vi "MNIST_Classifier_MLP(Train).vi.vi"() -> ()   [LabVIEW 2024]
doc: "This example demonstrating the usage of Deep Learning Toolkit for solving hand written digit recognition problem with multilayer perceptron (MLP).\nDataset: MNIST http://yann.lecun.com/exdb/mnist/\nRequirements: Deep Learning Toolkit for LabVIEW.s"
uses:
  <vilib>/Ngene/Deep Learning Toolkit/Toolkit/NN_Train/Controls/NN_Train_Params.ctl
  <vilib>/Ngene/Deep Learning Toolkit/Toolkit/NN_Train/Controls/NN_Train_Optimizer.ctl
  <vilib>/Ngene/Deep Learning Toolkit/Toolkit/NN_Train/Controls/NN_Train_Data_Sampling.ctl
  _Controls/Img_GrayScale.ctl
  <vilib>/Ngene/Deep Learning Toolkit/Toolkit/NN_Train/Controls/NN_Train_Session_Data.ctl
  <vilib>/Ngene/Deep Learning Toolkit/Toolkit/NN_Train/Controls/NN_LR_Policy_Cfg.ctl
  <vilib>/Ngene/Deep Learning Toolkit/Toolkit/NN_Train/Controls/NN_LR_Policy_Type.ctl
  <vilib>/Ngene/Deep Learning Toolkit/Toolkit/NN_Network/Controls/NN_Device.ctl
  <vilib>/Ngene/Deep Learning Toolkit/Toolkit/NN_Layers/Layers/FC/Controls/NN_Layer_Config(FC).ctl
  <vilib>/Ngene/Deep Learning Toolkit/Toolkit/NN_Layers/Layers/BatchNorm/Controls/NN_BN_Params.ctl
  <vilib>/Ngene/Deep Learning Toolkit/Toolkit/NN_Activations/Controls/NN_Activation_Type.ctl
  <vilib>/Ngene/Deep Learning Toolkit/Toolkit/NN_Layers/Controls/NN_Layer_Init_Params.ctl
  <vilib>/Ngene/Deep Learning Toolkit/Toolkit/NN_Layers/Controls/NN_Layer_Weight_Init_Type.ctl
  <vilib>/Ngene/Deep Learning Toolkit/Toolkit/NN_Layers/Layers/Input/Controls/NN_Layer_Config(Input1D).ctl
  <vilib>/Ngene/Deep Learning Toolkit/Toolkit/NN_Data/Controls/NN_Data_type.ctl
  <vilib>/Ngene/Deep Learning Toolkit/Toolkit/NN_Layers/Layers/DropOut3D/Controls/NN_Layer_Config(DropOut3D).ctl
  <vilib>/Ngene/Deep Learning Toolkit/Toolkit/NN_Network/Controls/NN_Save_Before_Destroy_Options.ctl
  <vilib>/Ngene/Deep Learning Toolkit/Toolkit/NN_Layers/Layers/Input/NN_Layer_Create(Input1D).vi
  <vilib>/Ngene/Deep Learning Toolkit/Toolkit/NN_Layers/Layers/FC/NN_Layer_Create(FC).vi
  <vilib>/Ngene/Deep Learning Toolkit/Toolkit/NN_Layers/Layers/Dropout/NN_Layer_Create(DropOut).vi
  <vilib>/Ngene/Deep Learning Toolkit/Toolkit/NN_Layers/Layers/SoftMax/NN_Layer_Create(SoftMax).vi
  <vilib>/Ngene/Deep Learning Toolkit/Toolkit/NN_Train/Loss_Functions/NN_Set_Loss(CrossEntropy).vi
  <vilib>/ptbypt/Filters.llb/FIR Filter PtByPt.vi
  <vilib>/Ngene/Deep Learning Toolkit/Toolkit/NN_Network/subVIs/NN_Predict/NN_Predict(In1D_Out1D).vi
  <vilib>/Ngene/Deep Learning Toolkit/Toolkit/NN_Train/Eval_Loss/NN_Eval_Test_Error_Loss/NN_Eval(In1D_Out1D).vi
  <vilib>/Ngene/Deep Learning Toolkit/Toolkit/NN_Train/Eval_Loss/NN_Calc_Cofusion_Matrix/NN_Calc_Confusion_Matrix(In1D_Out1D).vi
  <vilib>/Ngene/Deep Learning Toolkit/Toolkit/NN_Data/subVIs/Dataset_Destroy/NN_Datasets_All_Destroy(In1D_Out1D).vi
  <vilib>/Ngene/Deep Learning Toolkit/Toolkit/NN_Network/API/NN_Set_Input/1D/NN_Set_Input(1D_SGL_idx).vi
  <vilib>/Ngene/Deep Learning Toolkit/Toolkit/Deep_Learning_Toolkit_by_Ngene.lvlib
panel:
  in  "Tab":T1(tab)
  in  "NN_Device":T2
  out "Train Speed (img/s)":dbl=20473.778145437056 format="%#_2p"
  out "Train Graphs":T3(graph)
  in  "Check_Vald":bool
  out "Session Data":T4={"Epochs"=3.8804212, "Tot_Iter"=1728, "LR"=0.03001, "LR_iter"=1729}
  in  "Stop_Train":bool
  out "Train/Val_Metrics":T5={"Train_Loss"=0.05827807, "Valid_Loss"=0.04526825, "Valid_Error"=0.042666666} {"Train_Loss" format="%#_4g"; "Valid_Loss" format="%#_3g"}
  in  "LR Update Policy":T6={"Policy_Type"=enum."Step", "LR0"=0.03000999999873693, "k"=10.0, "WarmUp_Policy"=enum."Step", "WarmUp_Iter"=1, "WarmUp_Ratio"=1.0} {"WarmUp_Ratio" min=1; "WarmUp_Iter" min=1; "LR0" format="%.7f"}
  out "Train Speed (s/iter)":dbl=0.006251899336348288 format="%#_2p"
  in  "Train_Params":T8={"Optimizer"=enum."SGD", "Beta_1"=0.9, "Beta_2"=0.999, "Weight Decay(L1)"=1e-08, "Weight Decay(L2)"=1e-08, "Data_Sampling"=enum."Random"}
  out "Time_Elapsed":dbl=10.654257025802508 format="%<%H:%M:%S>t"
  out "Test_Loss":sgl=0.12478909 format="%#_3g"
  out "Test_Error":sgl=0.0388
  in  "Working Dir":path=path "D:/working"
  in  "MNIST Dataset Path":path
  out "Labels":string[](array[string])=["0", "1", "2", "3", "4", "5", "6", "7", "8", "9"]
  out "Draw Digit (280x280 px)":picture
  in  "Pen Color":u32(colorbox)=197379
  in  "Clear":bool
  out "Test Speed (img/s)":dbl=743.0102790718987 format="%#_2p"
  out "test time(s/img)":dbl=0.0013458764005918056 format="%#_3p"
  out "Predictions":sgl[](array[slide])=[0.00022317072, 0.0016224136, 0.00590554, 0.9895844, 0.0010204009, 0.00023260966, 0.00083900435, 0.00020435848, 0.00020539068, 0.00016265694] scale=0.0..1.0
  in  "Pen Width":u16=26
  in  "Stop Test":bool
  out "Pen Attributes":T11={"Width"=26, "Style"=enum."Solid"}
  out "image (28x28px)":sgl[][](graph)=[[-1.0, -1.0, -1.0, -1.0, -1.0, -1.0, -1.0, -1.0, -1.0, -1.0, -1.0, -1.0, -1.0, -1.0, -1.0, -1.0, -1.0, -1.0, -1.0, -1.0, -1.0, -1.0, -1.0, -1.0, -1.0, -1.0, -1.0, -1.0], [-1.0, -1.0, -1.0, -1.0, -1.0, -1.0, -1.0, -1.0, -0.97637796, -0.33858266, 0.32283464, 0.6062992, 0.6062992, 0.32283464, -0.19685039, -0.96062994, -1.0, -1.0, -1.0, -1.0, -1.0, -1.0, -1.0, -1.0, -1.0, -1.0, -1.0, -1.0], [-1.0, -1.0, -1.0, -1.0, -1.0, -1.0, -1.0, -0.8976378, 0.503937, 1.007874, 1.007874, 1.007874, 1.007874, 1.007874, 1.007874, 0.5826772, -0.97637796, -1.0, -1.0, -1.0, -1.0, -1.0, -1.0, -1.0, -1.0, -1.0, -1.0, -1.0], [-1.0, -1.0, -1.0, -1.0, -1.0, -1.0, -1.0, 0.047244094, 1.007874, 1.007874, 1.007874, 0.68503934, 0.62992126, 0.9448819, 1.007874, 1.007874, 0.12598425, -1.0, -1.0, -1.0, -1.0, -1.0, -1.0, -1.0, -1.0, -1.0, -1.0, -1.0], [-1.0, -1.0, -1.0, -1.0, -1.0, -1.0, -1.0, 0.8267717, 1.007874, 0.9055118, -0.77952754, -1.0, -1.0, -0.79527557, 0.8267717, 1.007874, 0.86614174, -1.0, -1.0, -1.0, -1.0, -1.0, -1.0, -1.0, -1.0, -1.0, -1.0, -1.0], [-1.0, -1.0, -1.0, -1.0, -1.0, -1.0, -0.79527557, 1.007874, 1.007874, 0.16535433, -1.0, -1.0, -1.0, -1.0, 0.22834645, 1.007874, 1.007874, -1.0, -1.0, -1.0, -1.0, -1.0, -1.0, -1.0, -1.0, -1.0, -1.0, -1.0], [-1.0, -1.0, -1.0, -1.0, -1.0, -1.0, -0.79527557, 1.007874, 1.007874, 0.007874016, -1.0, -1.0, -1.0, -1.0, 0.20472442, 1.007874, 1.007874, -1.0, -1.0, -1.0, -1.0, -1.0, -1.0, -1.0, -1.0, -1.0, -1.0, -1.0], [-1.0, -1.0, -1.0, -1.0, -1.0, -1.0, -0.8976378, 0.984252, 1.007874, 0.4015748, -1.0, -1.0, -1.0, -1.0, 0.20472442, 1.007874, 1.007874, -0.8582677, -1.0, -1.0, -1.0, -1.0, -1.0, -1.0, -1.0, -1.0, -1.0, -1.0], [-1.0, -1.0, -1.0, -1.0, -1.0, -1.0, -1.0, 0.56692916, 1.007874, 0.96850395, -0.6614173, -1.0, -1.0, -1.0, 0.503937, 1.007874, 1.007874, -0.96062994, -1.0, -1.0, -1.0, -1.0, -1.0, -1.0, -1.0, -1.0, -1.0, -1.0], [-1.0, -1.0, -1.0, -1.0, -1.0, -1.0, -1.0, -0.37795275, 1.007874, 1.007874, 0.7480315, -0.6771653, -1.0, -0.9212598, 0.96850395, 1.007874, 0.8110236, -1.0, -1.0, -1.0, -1.0, -1.0, -1.0, -1.0, -1.0, -1.0, -1.0, -1.0], [-1.0, -1.0, -1.0, -1.0, -1.0, -1.0, -1.0, -1.0, 0.3464567, 1.007874, 1.007874, 0.8897638, -0.31496063, -0.05511811, 1.007874, 1.007874, 0.24409449, -1.0, -1.0, -1.0, -1.0, -1.0, -1.0, -1.0, -1.0, -1.0, -1.0, -1.0], [-1.0, -1.0, -1.0, -1.0, -1.0, -1.0, -1.0, -1.0, -0.96062994, 0.26771653, 1.007874, 1.007874, 0.984252, 0.9055118, 1.007874, 0.9055118, -0.81889766, -1.0, -1.0, -1.0, -1.0, -1.0, -1.0, -1.0, -1.0, -1.0, -1.0, -1.0], [-1.0, -1.0, -1.0, -1.0, -1.0, -1.0, -1.0, -1.0, -1.0, -1.0, -0.15748031, 0.9448819, 1.007874, 1.007874, 1.007874, 0.36220473, -1.0, -1.0, -1.0, -1.0, -1.0, -1.0, -1.0, -1.0, -1.0, -1.0, -1.0, -1.0], [-1.0, -1.0, -1.0, -1.0, -1.0, -1.0, -1.0, -1.0, -1.0, -1.0, -1.0, -0.03937008, 1.007874, 1.007874, 1.007874, 1.007874, 0.30708662, -0.8582677, -1.0, -1.0, -1.0, -1.0, -1.0, -1.0, -1.0, -1.0, -1.0, -1.0], [-1.0, -1.0, -1.0, -1.0, -1.0, -1.0, -1.0, -1.0, -1.0, -1.0, -0.25984251, 0.92913383, 1.007874, 1.007874, 1.007874, 1.007874, 1.007874, 0.8110236, -0.77952754, -1.0, -1.0, -1.0, -1.0, -1.0, -1.0, -1.0, -1.0, -1.0], [-1.0, -1.0, -1.0, -1.0, -1.0, -1.0, -1.0, -1.0, -1.0, 0.047244094, 1.007874, 1.007874, 1.007874, 0.10236221, -0.5748032, 0.5826772, 1.007874, 1.007874, 0.08661418, -1.0, -1.0, -1.0, -1.0, -1.0, -1.0, -1.0, -1.0, -1.0], [-1.0, -1.0, -1.0, -1.0, -1.0, -1.0, -1.0, -1.0, -0.17322835, 1.007874, 1.007874, 0.9448819, -0.23622048, -1.0, -1.0, -0.8976378, 0.8267717, 1.007874, 0.92913383, -0.8425197, -1.0, -1.0, -1.0, -1.0, -1.0, -1.0, -1.0, -1.0], [-1.0, -1.0, -1.0, -1.0, -1.0, -1.0, -1.0, -1.0, 0.8503937, 1.007874, 0.9055118, -0.4015748, -1.0, -1.0, -1.0, -1.0, -0.07874016, 1.007874, 1.007874, -0.27559054, -1.0, -1.0, -1.0, -1.0, -1.0, -1.0, -1.0, -1.0], [-1.0, -1.0, -1.0, -1.0, -1.0, -1.0, -1.0, -0.44094488, 1.007874, 1.007874, 0.28346458, -1.0, -1.0, -1.0, -1.0, -1.0, -0.6771653, 1.007874, 1.007874, 0.16535433, -1.0, -1.0, -1.0, -1.0, -1.0, -1.0, -1.0, -1.0], [-1.0, -1.0, -1.0, -1.0, -1.0, -1.0, -1.0, 0.007874016, 1.007874, 1.007874, -0.5984252, -1.0, -1.0, -1.0, -1.0, -1.0, -0.79527557, 1.007874, 1.007874, 0.007874016, -1.0, -1.0, -1.0, -1.0, -1.0, -1.0, -1.0, -1.0], [-1.0, -1.0, -1.0, -1.0, -1.0, -1.0, -1.0, 0.007874016, 1.007874, 1.007874, -0.7401575, -1.0, -1.0, -1.0, -1.0, -1.0, -0.77952754, 1.007874, 1.007874, 0.007874016, -1.0, -1.0, -1.0, -1.0, -1.0, -1.0, -1.0, -1.0], [-1.0, -1.0, -1.0, -1.0, -1.0, -1.0, -1.0, -0.19685039, 1.007874, 1.007874, -0.5590551, -1.0, -1.0, -1.0, -1.0, -1.0, 0.14173229, 1.007874, 1.007874, -0.11811024, -1.0, -1.0, -1.0, -1.0, -1.0, -1.0, -1.0, -1.0], [-1.0, -1.0, -1.0, -1.0, -1.0, -1.0, -1.0, -0.496063, 1.007874, 1.007874, 0.023622047, -1.0, -1.0, -1.0, -0.7559055, 0.36220473, 1.007874, 1.007874, 0.86614174, -0.8582677, -1.0, -1.0, -1.0, -1.0, -1.0, -1.0, -1.0, -1.0], [-1.0, -1.0, -1.0, -1.0, -1.0, -1.0, -1.0, -0.96062994, 0.8503937, 1.007874, 0.9448819, 0.08661418, 0.007874016, 0.18110237, 0.92913383, 1.007874, 1.007874, 0.9055118, -0.51968503, -1.0, -1.0, -1.0, -1.0, -1.0, -1.0, -1.0, -1.0, -1.0], [-1.0, -1.0, -1.0, -1.0, -1.0, -1.0, -1.0, -1.0, -0.2992126, 1.007874, 1.007874, 1.007874, 1.007874, 1.007874, 1.007874, 1.007874, 0.62992126, -0.62204725, -1.0, -1.0, -1.0, -1.0, -1.0, -1.0, -1.0, -1.0, -1.0, -1.0], [-1.0, -1.0, -1.0, -1.0, -1.0, -1.0, -1.0, -1.0, -1.0, -0.11811024, 0.96850395, 1.007874, 1.007874, 1.007874, 0.68503934, -0.31496063, -1.0, -1.0, -1.0, -1.0, -1.0, -1.0, -1.0, -1.0, -1.0, -1.0, -1.0, -1.0], [-1.0, -1.0, -1.0, -1.0, -1.0, -1.0, -1.0, -1.0, -1.0, -1.0, -0.88188976, -0.79527557, -0.79527557, -0.88188976, -1.0, -1.0, -1.0, -1.0, -1.0, -1.0, -1.0, -1.0, -1.0, -1.0, -1.0, -1.0, -1.0, -1.0], [-1.0, -1.0, -1.0, -1.0, -1.0, -1.0, -1.0, -1.0, -1.0, -1.0, -1.0, -1.0, -1.0, -1.0, -1.0, -1.0, -1.0, -1.0, -1.0, -1.0, -1.0, -1.0, -1.0, -1.0, -1.0, -1.0, -1.0, -1.0]]
  out "Incorrectly Classified Imgs":T12[][](array[typedef])=[[{"image"=array28x28[784 elements], "Truth"=2, "Predicted"=2}, {"image"=array28x28[784 elements], "Truth"=9, "Predicted"=9}, {"image"=array28x28[784 elements], "Truth"=2, "Predicted"=2}, {"image"=array28x28[784 elements], "Truth"=7, "Predicted"=7}, {"image"=array28x28[784 elements], "Truth"=8, "Predicted"=8}, {"image"=array28x28[784 elements], "Truth"=2, "Predicted"=2}, {"image"=array28x28[784 elements], "Truth"=0, "Predicted"=0}, {"image"=array28x28[784 elements], "Truth"=1, "Predicted"=1}, {"image"=array28x28[784 elements], "Truth"=7, "Predicted"=7}, {"image"=array28x28[784 elements], "Truth"=3, "Predicted"=3}], [{"image"=array28x28[784 elements], "Truth"=7, "Predicted"=7}, {"image"=array28x28[784 elements], "Truth"=7, "Predicted"=7}, {"image"=array28x28[784 elements], "Truth"=7, "Predicted"=7}, {"image"=array28x28[784 elements], "Truth"=7, "Predicted"=7}, {"image"=array28x28[784 elements], "Truth"=0, "Predicted"=0}, {"image"=array28x28[784 elements], "Truth"=5, "Predicted"=5}, {"image"=array28x28[784 elements], "Truth"=2, "Predicted"=2}, {"image"=array28x28[784 elements], "Truth"=5, "Predicted"=5}, {"image"=array28x28[784 elements], "Truth"=8, "Predicted"=8}, {"image"=array28x28[784 elements], "Truth"=5, "Predicted"=5}], [{"image"=array28x28[784 elements], "Truth"=1, "Predicted"=1}, {"image"=array28x28[784 elements], "Truth"=9, "Predicted"=9}, {"image"=array28x28[784 elements], "Truth"=7, "Predicted"=7}, {"image"=array28x28[784 elements], "Truth"=2, "Predicted"=2}, {"image"=array28x28[784 elements], "Truth"=3, "Predicted"=3}, {"image"=array28x28[784 elements], "Truth"=9, "Predicted"=9}, {"image"=array28x28[784 elements], "Truth"=2, "Predicted"=2}, {"image"=array28x28[784 elements], "Truth"=7, "Predicted"=7}, {"image"=array28x28[784 elements], "Truth"=8, "Predicted"=8}, {"image"=array28x28[784 elements], "Truth"=4, "Predicted"=4}], [{"image"=array28x28[784 elements], "Truth"=0, "Predicted"=0}, {"image"=array28x28[784 elements], "Truth"=8, "Predicted"=8}, {"image"=array28x28[784 elements], "Truth"=3, "Predicted"=3}, {"image"=array28x28[784 elements], "Truth"=4, "Predicted"=4}, {"image"=array28x28[784 elements], "Truth"=9, "Predicted"=9}, {"image"=array28x28[784 elements], "Truth"=6, "Predicted"=6}, {"image"=array28x28[784 elements], "Truth"=9, "Predicted"=9}, {"image"=array28x28[784 elements], "Truth"=9, "Predicted"=9}, {"image"=array28x28[784 elements], "Truth"=5, "Predicted"=5}, {"image"=array28x28[784 elements], "Truth"=9, "Predicted"=9}], [{"image"=array28x28[784 elements], "Truth"=3, "Predicted"=3}, {"image"=array28x28[784 elements], "Truth"=7, "Predicted"=7}, {"image"=array28x28[784 elements], "Truth"=9, "Predicted"=9}, {"image"=array28x28[784 elements], "Truth"=7, "Predicted"=7}, {"image"=array28x28[784 elements], "Truth"=3, "Predicted"=3}, {"image"=array28x28[784 elements], "Truth"=7, "Predicted"=7}, {"image"=array28x28[784 elements], "Truth"=5, "Predicted"=5}, {"image"=array28x28[784 elements], "Truth"=7, "Predicted"=7}, {"image"=array28x28[784 elements], "Truth"=6, "Predicted"=6}, {"image"=array28x28[784 elements], "Truth"=9, "Predicted"=9}], [{"image"=array28x28[784 elements], "Truth"=0, "Predicted"=0}, {"image"=array28x28[784 elements], "Truth"=9, "Predicted"=9}, {"image"=array28x28[784 elements], "Truth"=2, "Predicted"=2}, {"image"=array28x28[784 elements], "Truth"=9, "Predicted"=9}, {"image"=array28x28[784 elements], "Truth"=5, "Predicted"=5}, {"image"=array28x28[784 elements], "Truth"=1, "Predicted"=1}, {"image"=array28x28[784 elements], "Truth"=8, "Predicted"=8}, {"image"=array28x28[784 elements], "Truth"=7, "Predicted"=7}, {"image"=array28x28[784 elements], "Truth"=4, "Predicted"=4}, {"image"=array28x28[784 elements], "Truth"=0, "Predicted"=0}], [{"image"=array28x28[784 elements], "Truth"=8, "Predicted"=8}, {"image"=array28x28[784 elements], "Truth"=6, "Predicted"=6}, {"image"=array28x28[784 elements], "Truth"=8, "Predicted"=8}, {"image"=array28x28[784 elements], "Truth"=1, "Predicted"=1}, {"image"=array28x28[784 elements], "Truth"=7, "Predicted"=7}, {"image"=array28x28[784 elements], "Truth"=7, "Predicted"=7}, {"image"=array28x28[784 elements], "Truth"=7, "Predicted"=7}, {"image"=array28x28[784 elements], "Truth"=2, "Predicted"=2}, {"image"=array28x28[784 elements], "Truth"=2, "Predicted"=2}, {"image"=array28x28[784 elements], "Truth"=4, "Predicted"=4}], [{"image"=array28x28[784 elements], "Truth"=5, "Predicted"=5}, {"image"=array28x28[784 elements], "Truth"=6, "Predicted"=6}, {"image"=array28x28[784 elements], "Truth"=1, "Predicted"=1}, {"image"=array28x28[784 elements], "Truth"=9, "Predicted"=9}, {"image"=array28x28[784 elements], "Truth"=9, "Predicted"=9}, {"image"=array28x28[784 elements], "Truth"=7, "Predicted"=7}, {"image"=array28x28[784 elements], "Truth"=3, "Predicted"=3}, {"image"=array28x28[784 elements], "Truth"=2, "Predicted"=2}, {"image"=array28x28[784 elements], "Truth"=6, "Predicted"=6}, {"image"=array28x28[784 elements], "Truth"=3, "Predicted"=3}], [{"image"=array28x28[784 elements], "Truth"=9, "Predicted"=9}, {"image"=array28x28[784 elements], "Truth"=5, "Predicted"=5}, {"image"=array28x28[784 elements], "Truth"=1, "Predicted"=1}, {"image"=array28x28[784 elements], "Truth"=0, "Predicted"=0}, {"image"=array28x28[784 elements], "Truth"=5, "Predicted"=5}, {"image"=array28x28[784 elements], "Truth"=7, "Predicted"=7}, {"image"=array28x28[784 elements], "Truth"=2, "Predicted"=2}, {"image"=array28x28[784 elements], "Truth"=5, "Predicted"=5}, {"image"=array28x28[784 elements], "Truth"=7, "Predicted"=7}, {"image"=array28x28[784 elements], "Truth"=4, "Predicted"=4}], [{"image"=array28x28[784 elements], "Truth"=9, "Predicted"=9}, {"image"=array28x28[784 elements], "Truth"=9, "Predicted"=9}, {"image"=array28x28[784 elements], "Truth"=5, "Predicted"=5}, {"image"=array28x28[784 elements], "Truth"=5, "Predicted"=5}, {"image"=array28x28[784 elements], "Truth"=3, "Predicted"=3}, {"image"=array28x28[784 elements], "Truth"=6, "Predicted"=6}, {"image"=array28x28[784 elements], "Truth"=7, "Predicted"=7}, {"image"=array28x28[784 elements], "Truth"=7, "Predicted"=7}, {"image"=array28x28[784 elements], "Truth"=7, "Predicted"=7}, {"image"=array28x28[784 elements], "Truth"=3, "Predicted"=3}], [{"image"=array28x28[784 elements], "Truth"=3, "Predicted"=3}, {"image"=array28x28[784 elements], "Truth"=7, "Predicted"=7}, {"image"=array28x28[784 elements], "Truth"=5, "Predicted"=5}, {"image"=array28x28[784 elements], "Truth"=3, "Predicted"=3}, {"image"=array28x28[784 elements], "Truth"=2, "Predicted"=2}, {"image"=array28x28[784 elements], "Truth"=5, "Predicted"=5}, {"image"=array28x28[784 elements], "Truth"=7, "Predicted"=7}, {"image"=array28x28[784 elements], "Truth"=9, "Predicted"=9}, {"image"=array28x28[784 elements], "Truth"=4, "Predicted"=4}, {"image"=array28x28[784 elements], "Truth"=5, "Predicted"=5}], [{"image"=array28x28[784 elements], "Truth"=9, "Predicted"=9}, {"image"=array28x28[784 elements], "Truth"=7, "Predicted"=7}, {"image"=array28x28[784 elements], "Truth"=5, "Predicted"=5}, {"image"=array28x28[784 elements], "Truth"=3, "Predicted"=3}, {"image"=array28x28[784 elements], "Truth"=0, "Predicted"=0}, {"image"=array28x28[784 elements], "Truth"=9, "Predicted"=9}, {"image"=array28x28[784 elements], "Truth"=4, "Predicted"=4}, {"image"=array28x28[784 elements], "Truth"=3, "Predicted"=3}, {"image"=array28x28[784 elements], "Truth"=4, "Predicted"=4}, {"image"=array28x28[784 elements], "Truth"=6, "Predicted"=6}], [{"image"=array28x28[784 elements], "Truth"=5, "Predicted"=5}, {"image"=array28x28[784 elements], "Truth"=5, "Predicted"=5}, {"image"=array28x28[784 elements], "Truth"=0, "Predicted"=0}, {"image"=array28x28[784 elements], "Truth"=9, "Predicted"=9}, {"image"=array28x28[784 elements], "Truth"=2, "Predicted"=2}, {"image"=array28x28[784 elements], "Truth"=3, "Predicted"=3}, {"image"=array28x28[784 elements], "Truth"=8, "Predicted"=8}, {"image"=array28x28[784 elements], "Truth"=7, "Predicted"=7}, {"image"=array28x28[784 elements], "Truth"=9, "Predicted"=9}, {"image"=array28x28[784 elements], "Truth"=9, "Predicted"=9}], [{"image"=array28x28[784 elements], "Truth"=0, "Predicted"=0}, {"image"=array28x28[784 elements], "Truth"=9, "Predicted"=9}, {"image"=array28x28[784 elements], "Truth"=7, "Predicted"=7}, {"image"=array28x28[784 elements], "Truth"=0, "Predicted"=0}, {"image"=array28x28[784 elements], "Truth"=2, "Predicted"=2}, {"image"=array28x28[784 elements], "Truth"=9, "Predicted"=9}, {"image"=array28x28[784 elements], "Truth"=1, "Predicted"=1}, {"image"=array28x28[784 elements], "Truth"=9, "Predicted"=9}, {"image"=array28x28[784 elements], "Truth"=5, "Predicted"=5}, {"image"=array28x28[784 elements], "Truth"=2, "Predicted"=2}], [{"image"=array28x28[784 elements], "Truth"=8, "Predicted"=8}, {"image"=array28x28[784 elements], "Truth"=5, "Predicted"=5}, {"image"=array28x28[784 elements], "Truth"=1, "Predicted"=1}, {"image"=array28x28[784 elements], "Truth"=6, "Predicted"=6}, {"image"=array28x28[784 elements], "Truth"=9, "Predicted"=9}, {"image"=array28x28[784 elements], "Truth"=6, "Predicted"=6}, {"image"=array28x28[784 elements], "Truth"=0, "Predicted"=0}, {"image"=array28x28[784 elements], "Truth"=7, "Predicted"=7}, {"image"=array28x28[784 elements], "Truth"=9, "Predicted"=9}, {"image"=array28x28[784 elements], "Truth"=9, "Predicted"=9}], [{"image"=array28x28[784 elements], "Truth"=7, "Predicted"=7}, {"image"=array28x28[784 elements], "Truth"=1, "Predicted"=1}, {"image"=array28x28[784 elements], "Truth"=5, "Predicted"=5}, {"image"=array28x28[784 elements], "Truth"=9, "Predicted"=9}, {"image"=array28x28[784 elements], "Truth"=3, "Predicted"=3}, {"image"=array28x28[784 elements], "Truth"=9, "Predicted"=9}, {"image"=array28x28[784 elements], "Truth"=4, "Predicted"=4}, {"image"=array28x28[784 elements], "Truth"=9, "Predicted"=9}, {"image"=array28x28[784 elements], "Truth"=9, "Predicted"=9}, {"image"=array28x28[784 elements], "Truth"=6, "Predicted"=6}], [{"image"=array28x28[784 elements], "Truth"=9, "Predicted"=9}, {"image"=array28x28[784 elements], "Truth"=2, "Predicted"=2}, {"image"=array28x28[784 elements], "Truth"=8, "Predicted"=8}, {"image"=array28x28[784 elements], "Truth"=8, "Predicted"=8}, {"image"=array28x28[784 elements], "Truth"=5, "Predicted"=5}, {"image"=array28x28[784 elements], "Truth"=1, "Predicted"=1}, {"image"=array28x28[784 elements], "Truth"=7, "Predicted"=7}, {"image"=array28x28[784 elements], "Truth"=0, "Predicted"=0}, {"image"=array28x28[784 elements], "Truth"=5, "Predicted"=5}, {"image"=array28x28[784 elements], "Truth"=9, "Predicted"=9}], [{"image"=array28x28[784 elements], "Truth"=5, "Predicted"=5}, {"image"=array28x28[784 elements], "Truth"=3, "Predicted"=3}, {"image"=array28x28[784 elements], "Truth"=0, "Predicted"=0}, {"image"=array28x28[784 elements], "Truth"=9, "Predicted"=9}, {"image"=array28x28[784 elements], "Truth"=2, "Predicted"=2}, {"image"=array28x28[784 elements], "Truth"=2, "Predicted"=2}, {"image"=array28x28[784 elements], "Truth"=5, "Predicted"=5}, {"image"=array28x28[784 elements], "Truth"=5, "Predicted"=5}, {"image"=array28x28[784 elements], "Truth"=3, "Predicted"=3}, {"image"=array28x28[784 elements], "Truth"=7, "Predicted"=7}], [{"image"=array28x28[784 elements], "Truth"=9, "Predicted"=9}, {"image"=array28x28[784 elements], "Truth"=9, "Predicted"=9}, {"image"=array28x28[784 elements], "Truth"=7, "Predicted"=7}, {"image"=array28x28[784 elements], "Truth"=8, "Predicted"=8}, {"image"=array28x28[784 elements], "Truth"=7, "Predicted"=7}, {"image"=array28x28[784 elements], "Truth"=3, "Predicted"=3}, {"image"=array28x28[784 elements], "Truth"=3, "Predicted"=3}, {"image"=array28x28[784 elements], "Truth"=6, "Predicted"=6}, {"image"=array28x28[784 elements], "Truth"=9, "Predicted"=9}, {"image"=array28x28[784 elements], "Truth"=0, "Predicted"=0}], [{"image"=array28x28[784 elements], "Truth"=2, "Predicted"=2}, {"image"=array28x28[784 elements], "Truth"=9, "Predicted"=9}, {"image"=array28x28[784 elements], "Truth"=9, "Predicted"=9}, {"image"=array28x28[784 elements], "Truth"=2, "Predicted"=2}, {"image"=array28x28[784 elements], "Truth"=0, "Predicted"=0}, {"image"=array28x28[784 elements], "Truth"=7, "Predicted"=7}, {"image"=array28x28[784 elements], "Truth"=9, "Predicted"=9}, {"image"=array28x28[784 elements], "Truth"=9, "Predicted"=9}, {"image"=array28x28[784 elements], "Truth"=7, "Predicted"=7}, {"image"=array28x28[784 elements], "Truth"=9, "Predicted"=9}], [{"image"=array28x28[784 elements], "Truth"=9, "Predicted"=9}, {"image"=array28x28[784 elements], "Truth"=9, "Predicted"=9}, {"image"=array28x28[784 elements], "Truth"=0, "Predicted"=0}, {"image"=array28x28[784 elements], "Truth"=9, "Predicted"=9}, {"image"=array28x28[784 elements], "Truth"=7, "Predicted"=7}, {"image"=array28x28[784 elements], "Truth"=9, "Predicted"=9}, {"image"=array28x28[784 elements], "Truth"=1, "Predicted"=1}, {"image"=array28x28[784 elements], "Truth"=7, "Predicted"=7}, {"image"=array28x28[784 elements], "Truth"=4, "Predicted"=4}, {"image"=array28x28[784 elements], "Truth"=2, "Predicted"=2}], [{"image"=array28x28[784 elements], "Truth"=5, "Predicted"=5}, {"image"=array28x28[784 elements], "Truth"=0, "Predicted"=0}, {"image"=array28x28[784 elements], "Truth"=5, "Predicted"=5}, {"image"=array28x28[784 elements], "Truth"=7, "Predicted"=7}, {"image"=array28x28[784 elements], "Truth"=3, "Predicted"=3}, {"image"=array28x28[784 elements], "Truth"=3, "Predicted"=3}, {"image"=array28x28[784 elements], "Truth"=3, "Predicted"=3}, {"image"=array28x28[784 elements], "Truth"=3, "Predicted"=3}, {"image"=array28x28[784 elements], "Truth"=9, "Predicted"=9}, {"image"=array28x28[784 elements], "Truth"=9, "Predicted"=9}], [{"image"=array28x28[784 elements], "Truth"=5, "Predicted"=5}, {"image"=array28x28[784 elements], "Truth"=2, "Predicted"=2}, {"image"=array28x28[784 elements], "Truth"=6, "Predicted"=6}, {"image"=array28x28[784 elements], "Truth"=8, "Predicted"=8}, {"image"=array28x28[784 elements], "Truth"=7, "Predicted"=7}, {"image"=array28x28[784 elements], "Truth"=1, "Predicted"=1}, {"image"=array28x28[784 elements], "Truth"=3, "Predicted"=3}, {"image"=array28x28[784 elements], "Truth"=6, "Predicted"=6}, {"image"=array28x28[784 elements], "Truth"=7, "Predicted"=7}, {"image"=array28x28[784 elements], "Truth"=1, "Predicted"=1}], [{"image"=array28x28[784 elements], "Truth"=0, "Predicted"=0}, {"image"=array28x28[784 elements], "Truth"=4, "Predicted"=4}, {"image"=array28x28[784 elements], "Truth"=3, "Predicted"=3}, {"image"=array28x28[784 elements], "Truth"=3, "Predicted"=3}, {"image"=array28x28[784 elements], "Truth"=6, "Predicted"=6}, {"image"=array28x28[784 elements], "Truth"=5, "Predicted"=5}, {"image"=array28x28[784 elements], "Truth"=1, "Predicted"=1}, {"image"=array28x28[784 elements], "Truth"=7, "Predicted"=7}, {"image"=array28x28[784 elements], "Truth"=9, "Predicted"=9}, {"image"=array28x28[784 elements], "Truth"=1, "Predicted"=1}], [{"image"=array28x28[784 elements], "Truth"=5, "Predicted"=5}, {"image"=array28x28[784 elements], "Truth"=9, "Predicted"=9}, {"image"=array28x28[784 elements], "Truth"=6, "Predicted"=6}, {"image"=array28x28[784 elements], "Truth"=0, "Predicted"=0}, {"image"=array28x28[784 elements], "Truth"=3, "Predicted"=3}, {"image"=array28x28[784 elements], "Truth"=3, "Predicted"=3}, {"image"=array28x28[784 elements], "Truth"=2, "Predicted"=2}, {"image"=array28x28[784 elements], "Truth"=1, "Predicted"=1}, {"image"=array28x28[784 elements], "Truth"=0, "Predicted"=0}, {"image"=array28x28[784 elements], "Truth"=7, "Predicted"=7}], [{"image"=array28x28[784 elements], "Truth"=5, "Predicted"=5}, {"image"=array28x28[784 elements], "Truth"=6, "Predicted"=6}, {"image"=array28x28[784 elements], "Truth"=5, "Predicted"=5}, {"image"=array28x28[784 elements], "Truth"=3, "Predicted"=3}, {"image"=array28x28[784 elements], "Truth"=7, "Predicted"=7}, {"image"=array28x28[784 elements], "Truth"=9, "Predicted"=9}, {"image"=array28x28[784 elements], "Truth"=0, "Predicted"=0}, {"image"=array28x28[784 elements], "Truth"=7, "Predicted"=7}, {"image"=array28x28[784 elements], "Truth"=6, "Predicted"=6}, {"image"=array28x28[784 elements], "Truth"=7, "Predicted"=7}], [{"image"=array28x28[784 elements], "Truth"=9, "Predicted"=9}, {"image"=array28x28[784 elements], "Truth"=6, "Predicted"=6}, {"image"=array28x28[784 elements], "Truth"=9, "Predicted"=9}, {"image"=array28x28[784 elements], "Truth"=4, "Predicted"=4}, {"image"=array28x28[784 elements], "Truth"=3, "Predicted"=3}, {"image"=array28x28[784 elements], "Truth"=7, "Predicted"=7}, {"image"=array28x28[784 elements], "Truth"=2, "Predicted"=2}, {"image"=array28x28[784 elements], "Truth"=2, "Predicted"=2}, {"image"=array28x28[784 elements], "Truth"=0, "Predicted"=0}, {"image"=array28x28[784 elements], "Truth"=7, "Predicted"=7}], [{"image"=array28x28[784 elements], "Truth"=7, "Predicted"=7}, {"image"=array28x28[784 elements], "Truth"=3, "Predicted"=3}, {"image"=array28x28[784 elements], "Truth"=1, "Predicted"=1}, {"image"=array28x28[784 elements], "Truth"=7, "Predicted"=7}, {"image"=array28x28[784 elements], "Truth"=5, "Predicted"=5}, {"image"=array28x28[784 elements], "Truth"=4, "Predicted"=4}, {"image"=array28x28[784 elements], "Truth"=9, "Predicted"=9}, {"image"=array28x28[784 elements], "Truth"=2, "Predicted"=2}, {"image"=array28x28[784 elements], "Truth"=9, "Predicted"=9}, {"image"=array28x28[784 elements], "Truth"=4, "Predicted"=4}], [{"image"=array28x28[784 elements], "Truth"=9, "Predicted"=9}, {"image"=array28x28[784 elements], "Truth"=3, "Predicted"=3}, {"image"=array28x28[784 elements], "Truth"=2, "Predicted"=2}, {"image"=array28x28[784 elements], "Truth"=7, "Predicted"=7}, {"image"=array28x28[784 elements], "Truth"=7, "Predicted"=7}, {"image"=array28x28[784 elements], "Truth"=4, "Predicted"=4}, {"image"=array28x28[784 elements], "Truth"=8, "Predicted"=8}, {"image"=array28x28[784 elements], "Truth"=0, "Predicted"=0}, {"image"=array28x28[784 elements], "Truth"=0, "Predicted"=0}, {"image"=array28x28[784 elements], "Truth"=4, "Predicted"=4}], [{"image"=array28x28[784 elements], "Truth"=2, "Predicted"=2}, {"image"=array28x28[784 elements], "Truth"=9, "Predicted"=9}, {"image"=array28x28[784 elements], "Truth"=0, "Predicted"=0}, {"image"=array28x28[784 elements], "Truth"=6, "Predicted"=6}, {"image"=array28x28[784 elements], "Truth"=5, "Predicted"=5}, {"image"=array28x28[784 elements], "Truth"=1, "Predicted"=1}, {"image"=array28x28[784 elements], "Truth"=5, "Predicted"=5}, {"image"=array28x28[784 elements], "Truth"=4, "Predicted"=4}, {"image"=array28x28[784 elements], "Truth"=7, "Predicted"=7}, {"image"=array28x28[784 elements], "Truth"=3, "Predicted"=3}], [{"image"=array28x28[784 elements], "Truth"=4, "Predicted"=4}, {"image"=array28x28[784 elements], "Truth"=1, "Predicted"=1}, {"image"=array28x28[784 elements], "Truth"=7, "Predicted"=7}, {"image"=array28x28[784 elements], "Truth"=2, "Predicted"=2}, {"image"=array28x28[784 elements], "Truth"=4, "Predicted"=4}, {"image"=array28x28[784 elements], "Truth"=9, "Predicted"=9}, {"image"=array28x28[784 elements], "Truth"=8, "Predicted"=8}, {"image"=array28x28[784 elements], "Truth"=3, "Predicted"=3}, {"image"=array28x28[784 elements], "Truth"=9, "Predicted"=9}, {"image"=array28x28[784 elements], "Truth"=9, "Predicted"=9}], [{"image"=array28x28[784 elements], "Truth"=4, "Predicted"=4}, {"image"=array28x28[784 elements], "Truth"=6, "Predicted"=6}, {"image"=array28x28[784 elements], "Truth"=9, "Predicted"=9}, {"image"=array28x28[784 elements], "Truth"=3, "Predicted"=3}, {"image"=array28x28[784 elements], "Truth"=5, "Predicted"=5}, {"image"=array28x28[784 elements], "Truth"=1, "Predicted"=1}, {"image"=array28x28[784 elements], "Truth"=5, "Predicted"=5}, {"image"=array28x28[784 elements], "Truth"=7, "Predicted"=7}, {"image"=array28x28[784 elements], "Truth"=5, "Predicted"=5}, {"image"=array28x28[784 elements], "Truth"=7, "Predicted"=7}], [{"image"=array28x28[784 elements], "Truth"=9, "Predicted"=9}, {"image"=array28x28[784 elements], "Truth"=0, "Predicted"=0}, {"image"=array28x28[784 elements], "Truth"=0, "Predicted"=0}, {"image"=array28x28[784 elements], "Truth"=3, "Predicted"=3}, {"image"=array28x28[784 elements], "Truth"=9, "Predicted"=9}, {"image"=array28x28[784 elements], "Truth"=8, "Predicted"=8}, {"image"=array28x28[784 elements], "Truth"=9, "Predicted"=9}, {"image"=array28x28[784 elements], "Truth"=5, "Predicted"=5}, {"image"=array28x28[784 elements], "Truth"=9, "Predicted"=9}, {"image"=array28x28[784 elements], "Truth"=9, "Predicted"=9}], [{"image"=array28x28[784 elements], "Truth"=5, "Predicted"=5}, {"image"=array28x28[784 elements], "Truth"=5, "Predicted"=5}, {"image"=array28x28[784 elements], "Truth"=5, "Predicted"=5}, {"image"=array28x28[784 elements], "Truth"=5, "Predicted"=5}, {"image"=array28x28[784 elements], "Truth"=5, "Predicted"=5}, {"image"=array28x28[784 elements], "Truth"=2, "Predicted"=2}, {"image"=array28x28[784 elements], "Truth"=6, "Predicted"=6}, {"image"=array28x28[784 elements], "Truth"=0, "Predicted"=0}, {"image"=array28x28[784 elements], "Truth"=7, "Predicted"=7}, {"image"=array28x28[784 elements], "Truth"=5, "Predicted"=5}], [{"image"=array28x28[784 elements], "Truth"=7, "Predicted"=7}, {"image"=array28x28[784 elements], "Truth"=7, "Predicted"=7}, {"image"=array28x28[784 elements], "Truth"=7, "Predicted"=7}, {"image"=array28x28[784 elements], "Truth"=5, "Predicted"=5}, {"image"=array28x28[784 elements], "Truth"=7, "Predicted"=7}, {"image"=array28x28[784 elements], "Truth"=5, "Predicted"=5}, {"image"=array28x28[784 elements], "Truth"=5, "Predicted"=5}, {"image"=array28x28[784 elements], "Truth"=9, "Predicted"=9}, {"image"=array28x28[784 elements], "Truth"=5, "Predicted"=5}, {"image"=array28x28[784 elements], "Truth"=9, "Predicted"=9}], [{"image"=array28x28[784 elements], "Truth"=4, "Predicted"=4}, {"image"=array28x28[784 elements], "Truth"=9, "Predicted"=9}, {"image"=array28x28[784 elements], "Truth"=7, "Predicted"=7}, {"image"=array28x28[784 elements], "Truth"=7, "Predicted"=7}, {"image"=array28x28[784 elements], "Truth"=7, "Predicted"=7}, {"image"=array28x28[784 elements], "Truth"=5, "Predicted"=5}, {"image"=array28x28[784 elements], "Truth"=7, "Predicted"=7}, {"image"=array28x28[784 elements], "Truth"=0, "Predicted"=0}, {"image"=array28x28[784 elements], "Truth"=2, "Predicted"=2}, {"image"=array28x28[784 elements], "Truth"=8, "Predicted"=8}], [{"image"=array28x28[784 elements], "Truth"=5, "Predicted"=5}, {"image"=array28x28[784 elements], "Truth"=7, "Predicted"=7}, {"image"=array28x28[784 elements], "Truth"=7, "Predicted"=7}, {"image"=array28x28[784 elements], "Truth"=3, "Predicted"=3}, {"image"=array28x28[784 elements], "Truth"=9, "Predicted"=9}, {"image"=array28x28[784 elements], "Truth"=9, "Predicted"=9}, {"image"=array28x28[784 elements], "Truth"=8, "Predicted"=8}, {"image"=array28x28[784 elements], "Truth"=8, "Predicted"=8}, {"image"=array28x28[784 elements], "Truth"=8, "Predicted"=8}, {"image"=array28x28[784 elements], "Truth"=2, "Predicted"=2}], [{"image"=array28x28[784 elements], "Truth"=2, "Predicted"=2}, {"image"=array28x28[784 elements], "Truth"=8, "Predicted"=8}, {"image"=array28x28[784 elements], "Truth"=9, "Predicted"=9}, {"image"=array28x28[784 elements], "Truth"=8, "Predicted"=8}, {"image"=array28x28[784 elements], "Truth"=6, "Predicted"=6}, {"image"=array28x28[784 elements], "Truth"=8, "Predicted"=8}, {"image"=array28x28[784 elements], "Truth"=8, "Predicted"=8}, {"image"=array28x28[784 elements], "Truth"=9, "Predicted"=9}, {"image"=array28x28[784 elements], "Truth"=5, "Predicted"=5}, {"image"=array28x28[784 elements], "Truth"=9, "Predicted"=9}], [{"image"=array28x28[784 elements], "Truth"=5, "Predicted"=5}, {"image"=array28x28[784 elements], "Truth"=5, "Predicted"=5}, {"image"=array28x28[784 elements], "Truth"=7, "Predicted"=7}, {"image"=array28x28[784 elements], "Truth"=4, "Predicted"=4}, {"image"=array28x28[784 elements], "Truth"=6, "Predicted"=6}, {"image"=array28x28[784 elements], "Truth"=9, "Predicted"=9}, {"image"=array28x28[784 elements], "Truth"=6, "Predicted"=6}, {"image"=array28x28[784 elements], "Truth"=6, "Predicted"=6}, {"image"=array28x28[784 elements], "Truth"=5, "Predicted"=5}, {"image"=array28x28[784 elements], "Truth"=9, "Predicted"=9}], [{"image"=array28x28[784 elements], "Truth"=6, "Predicted"=6}, {"image"=array28x28[784 elements], "Truth"=9, "Predicted"=9}, {"image"=array28x28[784 elements], "Truth"=2, "Predicted"=2}, {"image"=array28x28[784 elements], "Truth"=2, "Predicted"=2}, {"image"=array28x28[784 elements], "Truth"=2, "Predicted"=2}, {"image"=array28x28[784 elements], "Truth"=2, "Predicted"=2}, {"image"=array28x28[784 elements], "Truth"=8, "Predicted"=8}, {"image"=array28x28[784 elements], "Truth"=6, "Predicted"=6}, {"image"=array28x28[784 elements], "Truth"=9, "Predicted"=9}, {"image"=array28x28[784 elements], "Truth"=5, "Predicted"=5}], [{"image"=array28x28[784 elements], "Truth"=3, "Predicted"=3}, {"image"=array28x28[784 elements], "Truth"=2, "Predicted"=2}, {"image"=array28x28[784 elements], "Truth"=5, "Predicted"=5}, {"image"=array28x28[784 elements], "Truth"=4, "Predicted"=4}, {"image"=array28x28[784 elements], "Truth"=7, "Predicted"=7}, {"image"=array28x28[784 elements], "Truth"=7, "Predicted"=7}, {"image"=array28x28[784 elements], "Truth"=8, "Predicted"=8}, {"image"=array28x28[784 elements], "Truth"=7, "Predicted"=7}, {"image"=array28x28[784 elements], "Truth"=7, "Predicted"=7}, {"image"=array28x28[784 elements], "Truth"=5, "Predicted"=5}], [{"image"=array28x28[784 elements], "Truth"=2, "Predicted"=2}, {"image"=array28x28[784 elements], "Truth"=7, "Predicted"=7}, {"image"=array28x28[784 elements], "Truth"=7, "Predicted"=7}, {"image"=array28x28[784 elements], "Truth"=8, "Predicted"=8}, {"image"=array28x28[784 elements], "Truth"=0, "Predicted"=0}, {"image"=array28x28[784 elements], "Truth"=6, "Predicted"=6}, {"image"=array28x28[784 elements], "Truth"=7, "Predicted"=7}, {"image"=array28x28[784 elements], "Truth"=2, "Predicted"=2}, {"image"=array28x28[784 elements], "Truth"=0, "Predicted"=0}, {"image"=array28x28[784 elements], "Truth"=0, "Predicted"=0}], [{"image"=array28x28[784 elements], "Truth"=0, "Predicted"=0}, {"image"=array28x28[784 elements], "Truth"=0, "Predicted"=0}, {"image"=array28x28[784 elements], "Truth"=0, "Predicted"=0}, {"image"=array28x28[784 elements], "Truth"=7, "Predicted"=7}, {"image"=array28x28[784 elements], "Truth"=4, "Predicted"=4}, {"image"=array28x28[784 elements], "Truth"=3, "Predicted"=3}, {"image"=array28x28[784 elements], "Truth"=7, "Predicted"=7}, {"image"=array28x28[784 elements], "Truth"=5, "Predicted"=5}, {"image"=array28x28[784 elements], "Truth"=7, "Predicted"=7}, {"image"=array28x28[784 elements], "Truth"=6, "Predicted"=6}], [{"image"=array28x28[784 elements], "Truth"=0, "Predicted"=0}, {"image"=array28x28[784 elements], "Truth"=4, "Predicted"=4}, {"image"=array28x28[784 elements], "Truth"=9, "Predicted"=9}, {"image"=array28x28[784 elements], "Truth"=7, "Predicted"=7}, {"image"=array28x28[784 elements], "Truth"=2, "Predicted"=2}, {"image"=array28x28[784 elements], "Truth"=6, "Predicted"=6}, {"image"=array28x28[784 elements], "Truth"=5, "Predicted"=5}, {"image"=array28x28[784 elements], "Truth"=3, "Predicted"=3}, {"image"=array28x28[784 elements], "Truth"=2, "Predicted"=2}, {"image"=array28x28[784 elements], "Truth"=6, "Predicted"=6}]]
  out "Confusion Matrix":string[][](table)
  out "Valid_Error":sgl=0.025441667
  out "Valid_Loss":sgl=0.09893758
  in  "Stop_Test":bool
  # "7. Hit \"Stop Train\" button when Validation Loss/Errors are not decreasing any more (~20 epochs).\n8. Observe the Test Error value - this represents the final accuracy of the trained network.\n9. Go to the Testing tab.\n10. Draw some digit in Draw Digit Interface and observe correctness of the predictions in the Predictions  indicator. Observe testing speed.\n11. Stop the VI by pressing \"Stop Test\" button on Testing tab\n12. Go to the Incorrectly Classified Images tab and observe images that were incorrectly predicted by the network from the test dataset.\n13. Navigate to \"Confusion Matrix\" tab and observe the results on Test dataset.\n14. Observe the files generated at \"Working Dir\" directory. Navigate to Working directory. A directory with network name should have been created which should contain 3 files: model configuration file (.cfg), a file with trained weights (.bin), and a network visualization file (.svg) which can be opened in a web browser.\n15. Modify the network by changing network configuration on the block diagram. Go through the steps 3.-12. and observe influence on the test Loss/Error.\n16.(Optional) Change \"NN_Device\" value to \"GPU\" to compare execution speeds on GPU and CPU..\n\nMore Examples:  https://github.com/ngenehub/deepltk_examples"
  # "Overview: This example demonstrating the usage of Deep Learning Toolkit for solving hand written digit recognition problem with multilayer perceptron (MLP).\nDataset: MNIST http://yann.lecun.com/exdb/mnist/\nRequirements: Deep Learning Toolkit for LabVIEW.\nInstructions:\n1. Download MNIST dataset (4 files) from the link above and extract all files into one directory and provide the path to that directory at \"MNIST Dataset Path\" control.\n2. Set appropriate path at \"Working Dir\" control where the results of the training will be stored.\n3.  Run the VI with current configuration of the training parameters and Learning Rate update policy.\n4. Observe how the training loss is decreasing.\n5. Observe training speed.\n6. Periodically press \"Eval Validation\" button to evaluate Validation Loss/Error.\nNote that validation error evaluation influences the training speed, as the forward network inference is run for whole validation dataset."
  # "Displaying images from the dataset that were incorrectly classified by the trained network."
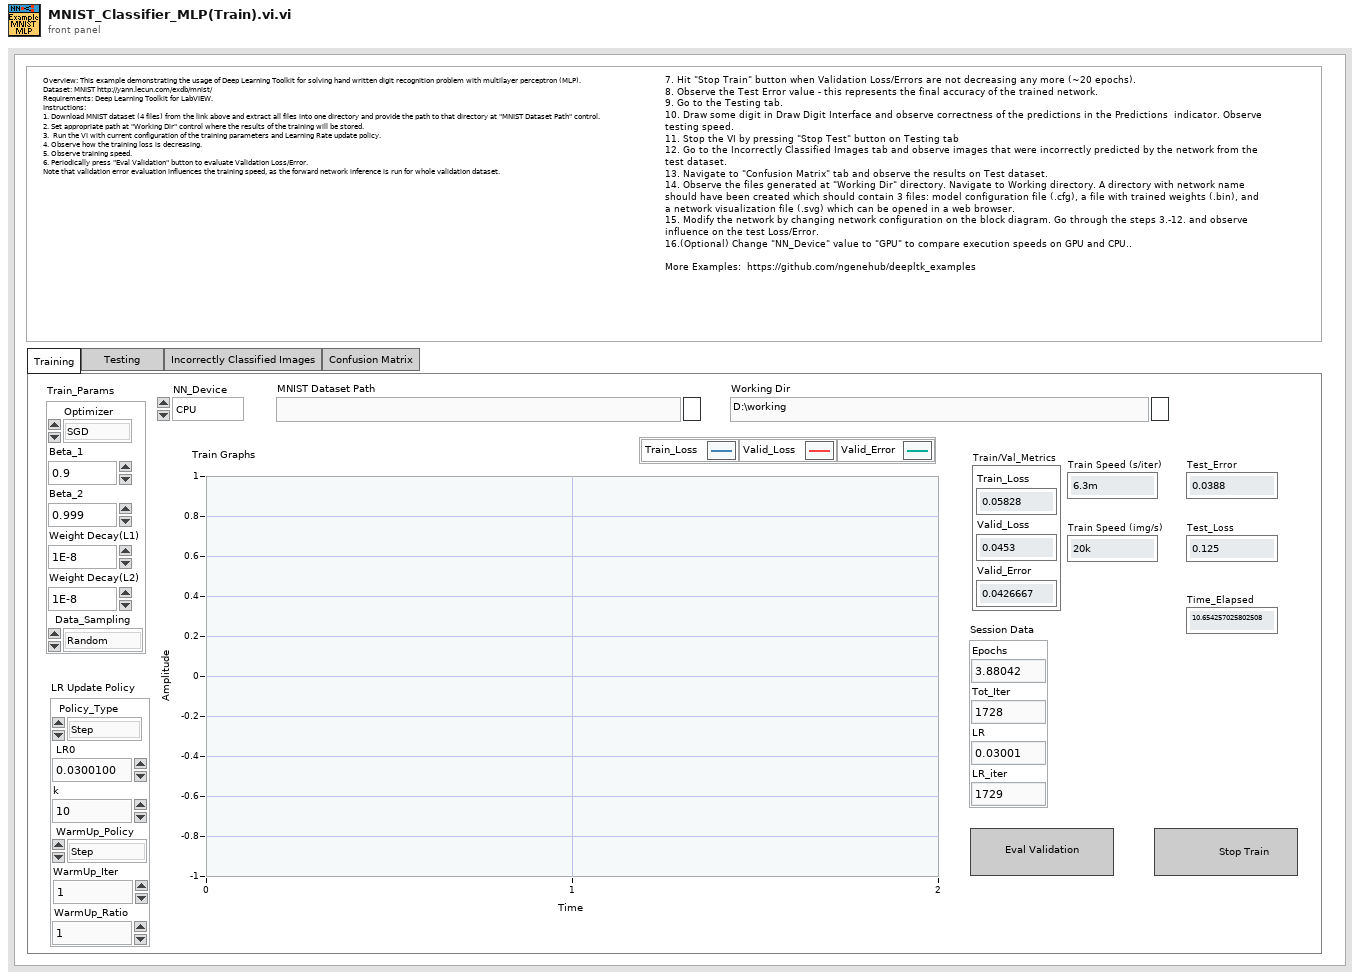
[diagram p1: front panel]
types:
  T1 = enum32{"Training", "Testing           ", "Incorrectly Classified Images", "Confusion Matrix"}
  T2 = typedef "Deep_Learning_Toolkit_by_Ngene.lvlib/NN_Device.ctl" = enum16{"CPU", "GPU"}
  T3 = cluster{"Filtered x":sgl, "Valid_Loss":sgl, "Valid_Error":sgl}
  T4 = typedef "Deep_Learning_Toolkit_by_Ngene.lvlib/NN_Train_Session_Data.ctl" = cluster{"Epochs":sgl, "Tot_Iter":i32, "LR":sgl, "LR_iter":i32}
  T5 = cluster{"Train_Loss":sgl, "Valid_Loss":sgl, "Valid_Error":sgl}
  T6 = typedef "Deep_Learning_Toolkit_by_Ngene.lvlib/NN_LR_Policy_Cfg.ctl" = cluster{"Policy_Type":T7, "LR0":dbl, "k":sgl, "WarmUp_Policy":enum16{"Step", "Ramp"}, "WarmUp_Iter":i32, "WarmUp_Ratio":sgl}
  T7 = typedef "Deep_Learning_Toolkit_by_Ngene.lvlib/NN_LR_Policy_Type.ctl" = enum16{"Manual", "Step", "Exp", "1/t"}
  T8 = typedef "Deep_Learning_Toolkit_by_Ngene.lvlib/NN_Train_Params.ctl" = cluster{"Optimizer":T9, "Beta_1":sgl, "Beta_2":sgl, "Weight Decay(L1)":sgl, "Weight Decay(L2)":sgl, "Data_Sampling":T10}
  T9 = typedef "Deep_Learning_Toolkit_by_Ngene.lvlib/NN_Train_Optimizer.ctl" = enum16{"SGD", "Adam", "Adagrad", "Adadelta", "RMSProp", "Nesterov"}
  T10 = typedef "Deep_Learning_Toolkit_by_Ngene.lvlib/NN_Train_Data_Sampling.ctl" = enum16{"Random", "Sequential"}
  T11 = cluster{"Width":u16, "Style":enum32{"Solid", "Dash", "Dot", "DashDot", "DashDotDot"}}
  T12 = typedef "Img_GrayScale.ctl" = cluster{"image":sgl[][], "Truth":i32, "Predicted":i32}
  T13 = typedef "Deep_Learning_Toolkit_by_Ngene.lvlib/NN_Layer_Config(FC).ctl" = cluster{"Name":string, "Size":i32, "BN":bool, "BN_Params":T14, "Activation":T15, "Has Bias?":bool, "Init_Params":T16, "Custom_Params":string}
  T14 = typedef "Deep_Learning_Toolkit_by_Ngene.lvlib/NN_BN_Params.ctl" = cluster{"epsilon":sgl, "momentum":sgl}
  T15 = typedef "Deep_Learning_Toolkit_by_Ngene.lvlib/NN_Activation_Type.ctl" = enum16{"Sigmoid", "ReLU", "LReLU", "ReLU6", "tanh", "Swish", "Mish", "None"}
  T16 = typedef "Deep_Learning_Toolkit_by_Ngene.lvlib/NN_Layer_Init_Params.ctl" = cluster{"Init_Type":T17, "Value":sgl}
  T17 = typedef "Deep_Learning_Toolkit_by_Ngene.lvlib/NN_Layer_Weight_Init_Type.ctl" = enum16{"Const", "Uniform", "Gaussian", "Xavier"}
  T18 = typedef "Deep_Learning_Toolkit_by_Ngene.lvlib/NN_Layer_Config(Input1D).ctl" = cluster{"Name":string, "Size":i32, "Data_Type":T19, "Shift":sgl, "Scale":sgl}
  T19 = typedef "Deep_Learning_Toolkit_by_Ngene.lvlib/NN_Data_type.ctl" = enum16{"I8", "U8", "I16", "U16", "U32 ARGB", "SGL"}
  T20 = typedef "Deep_Learning_Toolkit_by_Ngene.lvlib/NN_Layer_Config(DropOut3D).ctl" = cluster{"Name":string, "Probability":sgl}
  T21 = typedef "Deep_Learning_Toolkit_by_Ngene.lvlib/NN_Save_Before_Destroy_Options.ctl" = cluster{"CFG?":bool, "Weights?":bool, "Render?":bool}
  T22 = typedef "Deep_Learning_Toolkit_by_Ngene.lvlib/NN_DataSets_All(In1D_Out1D).ctl" = cluster{"Train":T23, "Validation":T23, "Test":T23}
  T23 = typedef "Deep_Learning_Toolkit_by_Ngene.lvlib/NN_DataSet(In1D_Out1D).ctl" = cluster{"Inputs Ref.":variant, "Outputs Ref.":T24, "Dims_In":i32, "Dataset_Size":i32, "Dims_Out":i32, "Labels":string[], "File Paths":path[]}
  T24 = typedef "Deep_Learning_Toolkit_by_Ngene.lvlib/NN_Data_ref(2D_SGL).ctl" = refnum<data-value>
  T25 = typedef "Deep_Learning_Toolkit_by_Ngene.lvlib/NN.ctl" = cluster{"Name":string, "No of Layers":i32, "mBatch":i32, "Layers":T26[], "Dimty":T27, "Dims_In":T28, "Dims_Out":T28, "Working_Dir":path, "Train?":bool, "Train_Params":T8, "LR_Update_Policy":T6, "Session Data":T4, "Ground_truth":T29, "NNg_hdls":T30, "NN_Device":T2, "GPU Id":i32, "Labels":string[], "Receptive Field":T31[], "Loss_Type":T32, "Loss_Cfg_Prms":variant, "NNG_WS":T33}
  T26 = typedef "Deep_Learning_Toolkit_by_Ngene.lvlib/NN_Layer_ref.ctl" = refnum<data-value>
  T27 = typedef "Deep_Learning_Toolkit_by_Ngene.lvlib/NN_In_Out_Dim-ty.ctl" = enum8{"In1D_Out1D", "In3D_Out1D", "In3D_Out3D", "In3D_OutBBox"}
  T28 = typedef "Deep_Learning_Toolkit_by_Ngene.lvlib/NN_Dims(C,H,W).ctl" = cluster{"C":i32, "H":i32, "W":i32}
  T29 = typedef "Deep_Learning_Toolkit_by_Ngene.lvlib/NN_Ground_truth.ctl" = cluster{"Y":variant}
  T30 = typedef "Deep_Learning_Toolkit_by_Ngene.lvlib/nng_cuda_handles.ctl" = cluster{"cudnn":u64, "cublas":u64, "stream":u64, "curand":u64}
  T31 = typedef "Deep_Learning_Toolkit_by_Ngene.lvlib/NN_Dims(V,H).ctl" = cluster{"V":i32, "H":i32}
  T32 = typedef "Deep_Learning_Toolkit_by_Ngene.lvlib/NN_Loss_Type.ctl" = enum16{"None", "MSE", "CrossEntropy", "YOLO_v2", "YOLO_v4"}
  T33 = typedef "Deep_Learning_Toolkit_by_Ngene.lvlib/NNG_WS.ctl" = cluster{"NNG_WS_Mem":T34, "Max_WS_Size":i64}
  T34 = typedef "Deep_Learning_Toolkit_by_Ngene.lvlib/NNg_WS_Mem_DVR.ctl" = refnum<data-value>
  T35 = typedef "Deep_Learning_Toolkit_by_Ngene.lvlib/NN_Eval_Params.ctl" = cluster{"Loss":sgl, "Error":sgl}
  T36 = typedef "Deep_Learning_Toolkit_by_Ngene.lvlib/NN_Layer.ctl" = cluster{"Name":string, "Layer_Data":variant, "Layer_Type":T37, "Dims_In":T28, "Layers_In":variant, "Dims_Out":T28, "Layers_Out":variant, "Metrics":T38, "GPU_Data":variant, "mBatch":i32, "NN_Device":T2, "NNg_hdls":T30, "Train?":bool, "Dimty":T39, "RecptField":T40}
  T37 = typedef "Deep_Learning_Toolkit_by_Ngene.lvlib/NN_Layer_Type.ctl" = enum16{"Input1D", "Input3D", "Conv1D", "Conv2D", "Conv2D_Adv", "MaxPool", "AvgPool", "UpSample", "DropOut3D", "ShortCut", "Concat", "SoftMax3D", "FC", "DropOut", "Softmax", "Flatten", "YOLO_v2", "YOLO_v4", "Activation", "BatchNormalization", "Unsupported"}
  T38 = typedef "Deep_Learning_Toolkit_by_Ngene.lvlib/NN_Layer_Metrics.ctl" = cluster{"Data":dbl, "Params":dbl, "Ops":dbl}
  T39 = typedef "Deep_Learning_Toolkit_by_Ngene.lvlib/NN_Layer_Dimty.ctl" = enum16{"1D", "3D"}
  T40 = typedef "Deep_Learning_Toolkit_by_Ngene.lvlib/NN_Layer_RF_State.ctl" = cluster{"Dims":T31, "J":T31}
  T41 = cluster{"left":i16, "top":i16, "right":i16, "bottom":i16}
  T42 = typedef "LVMouseTypeDef.ctl" = cluster{"Mouse Position":cluster{"X":i32, "Y":i32}, "Mouse Modifiers":cluster{"Button Down":bool, "Shift Mod":bool, "Menu Mod":bool, "Option Mod":bool}}
  T43 = typedef "imagedata.ctl" = cluster{"image type":i32, "image depth":i32, "image":u8[], "mask":u8[], "colors":u32[], "Rectangle":cluster{"left":i16, "top":i16, "right":i16, "bottom":i16}}
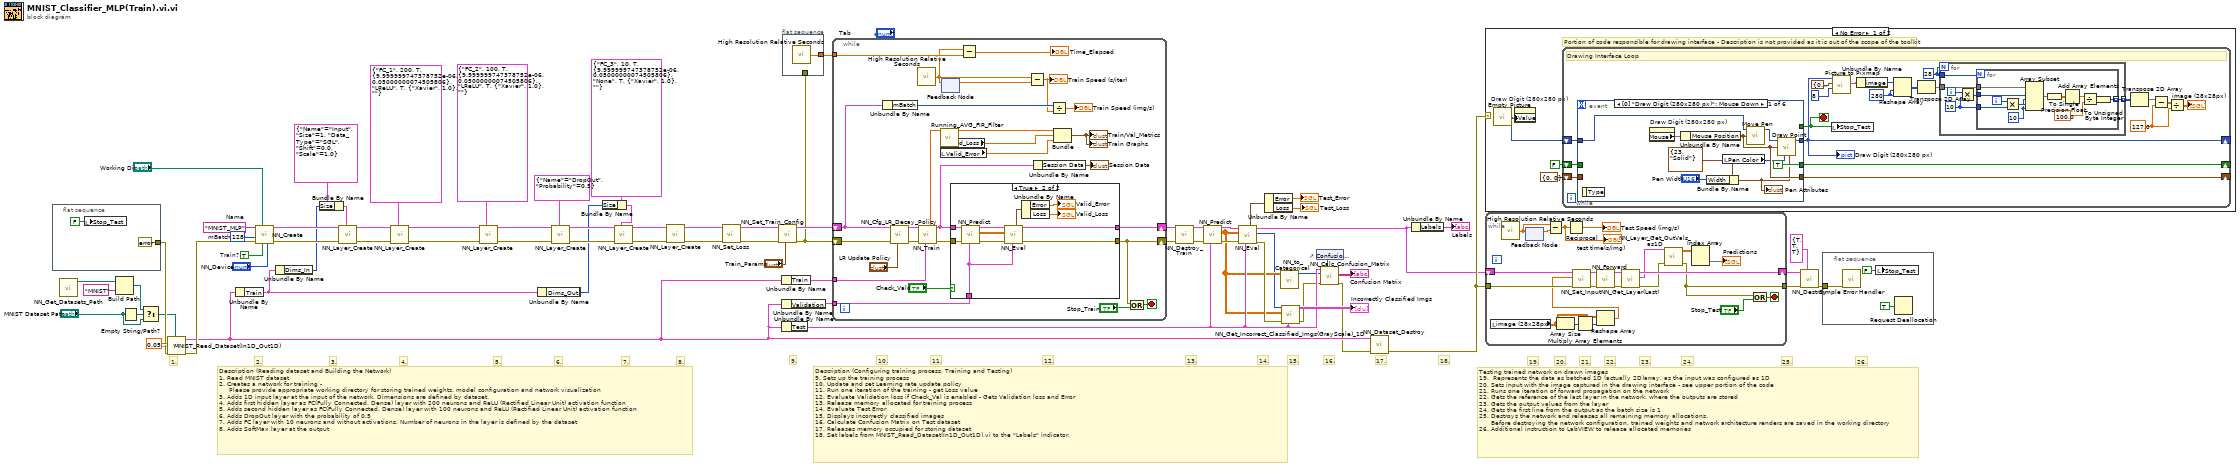
[diagram p0: block diagram]
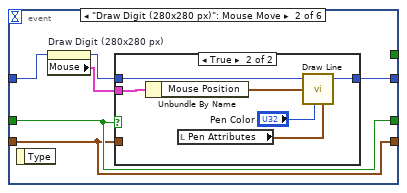
[diagram p3: hidden frame]
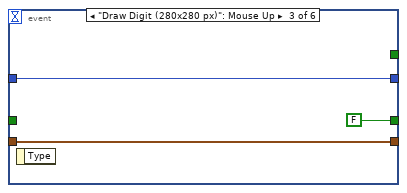
[diagram p5: hidden frame]
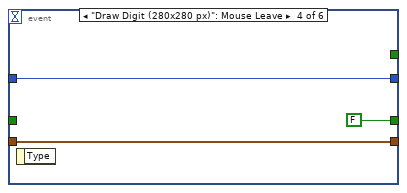
[diagram p6: hidden frame]
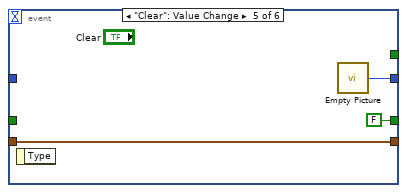
[diagram p7: hidden frame]
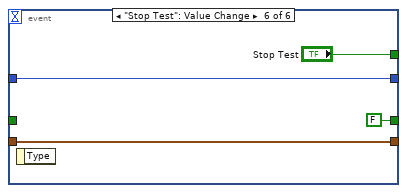
[diagram p8: hidden frame]
diagram:
  w47 = TRUE  # Train?
  w61 = 128  # mBatch
  w72 = "MNIST_MLP"  # Name
  # "26."
  # "25."
  # "Testing trained network on drawn images \n19.  Represents the data as batched 1D (actually 2D)array, as the input was configured as 1D\n20. Sets input with the image captured in the drawing interface - see upper portion of the code\n21. Runs one iteration of forward propagation on the network\n22. Gets the reference of the last layer in the network, where the outputs are stored\n23. Gets the output values from the layer\n24. Gets the first line from the output as the batch size is 1\n25. Destroys the network and releases all remaining memory allocations.\n      Before destroying the network configuration, trained weights and network architecture renders are saved in the working directory\n26. Additional instruction to LabVIEW to release allocated memories"
  # "24."
  # "23."
  # "22."
  # "21."
  # "20."
  # "19."
  # "18."
  # "16."
  # "Description (Configuring training process, Training and Testing)\n9. Sets up the training process\n10. Update and set Learning rate update policy\n11. Run one iteration of the training - get Loss value\n12. Evaluate Validation loss if Check_Val is enabled - Gets Validation loss and Error\n13. Release memory allocated for training process\n14. Evaluate Test Error\n15. Displays incorrectly classified images\n16. Calculate Confusion Matrix on Test dataset  \n17. Releases memory occupied for storing dataset\n18. Set labels from MNIST_Read_Dataset(In1D_Out1D).vi to the \"Labels\" indicator."
  # "17."
  # "15."
  # "14."
  # "13."
  # "12."
  # "11."
  # "10."
  # "9."
  # "Description (Reading dataset and Building the Network)\n1. Read MNIST dataset\n2. Creates a network for training - \n     Please provide appropriate working directory for storing trained weights, model configuration and network visualization\n3. Adds 1D input layer at the input of the network. Dimensions are defined by dataset.\n4. Adds first hidden layer as FC(Fully Connected, Dense) layer with 200 neurons and ReLU (Rectified Linear Unit) activation function\n5. Adds second hidden layer as FC(Fully Connected, Dense) layer with 100 neurons and ReLU (Rectified Linear Unit) activation function\n6. Adds DropOut layer with the probability of 0.5\n7. Adds FC layer with 10 neurons and without activations. Number of neurons in the layer is defined by the dataset\n8. Adds SoftMax layer at the output"
  # "8."
  # "7."
  # "6."
  # "5."
  # "4."
  # "3."
  # "2."
  # "1."
  n1 = flat-sequence {
    tunnel: [errorcluster {"status"=FALSE, "code"=0, "source"=""} ("error in (no error)")] -> w51
    frame #0 {
      n2 = local write "Stop_Test"(FALSE ("Stop_Test")) -> ()
    }
  }
  n3 = call "NN_Get_Datasets_Path.vi"() -> ("Datasets path"=w7:path)  [unwired: 11 in]
  n4 = Build Path(base path=w7, name or relative path="MNIST") -> (appended path=w9:path)
  n5 = Empty String/Path?(string/path="MNIST Dataset Path") -> (empty?=w8:bool)
  n6 = Select(t=w9, s=w8, f="MNIST Dataset Path") -> (s? t:f=w5:path)
  n7 = call "MNIST_Read_Dataset(In1D_Out1D).vi"("MNIST Dataset Path"=w5, "error in"=w51, "Validation_Size"=sgl 0.05 ("Valid_data_Size")) -> ("error out"=w73:errorcluster, "Datasets(Train,Val,Test)"=w29:T22)  [unwired: 7 in]
  n8 = Unbundle By Name(w29) -> ("Train"=w27:T23)
  n9 = call <vilib>:"NN_Create.vi"("NN_Device"="NN_Device", "Train? (false)"=w47, "Working Dir"="Working Dir", "error in (no error)"=w73, "mBatch (1)"=w61, "Name"=w72) -> ("error out"=w70:errorcluster, "NN out"=w71:T25)  [unwired: 4 in]
  n10 = Unbundle By Name(w27) -> ("Dims_In"=w28:i32)
  n11 = Bundle By Name(cluster=T18 {"Name"="Input", "Size"=1, "Data_Type"=enum."SGL", "Shift"=0.0, "Scale"=1.0} ("Input1D_Cfg"), "Size"=w28) -> (w31:T18)
  n12 = call-poly <vilib>:"NN_Layer_Create.vi"("Input1D_Cfg"=w31, "error in (no error)"=w70, "NN in"=w71) -> ("error out"=w56:errorcluster, "NN out"=w57:T25)  [unwired: 6 in, 1 out]
  n13 = call-poly <vilib>:"NN_Layer_Create.vi"("FC_Cfg"=T13 {"Name"="FC_1", "Size"=200, "BN"=TRUE, "BN_Params"={"epsilon"=1e-05, "momentum"=0.05}, "Activation"=enum."LReLU", "Has Bias?"=TRUE, "Init_Params"={"Init_Type"=enum."Xavier", "Value"=1.0}, "Custom_Params"=""} ("Layer_Config_Params"), "error in (no error)"=w56, "NN in"=w57) -> ("error out"=w43:errorcluster, "NN out"=w44:T25)  [unwired: 6 in, 1 out]
  n14 = call-poly <vilib>:"NN_Layer_Create.vi"("FC_Cfg"=T13 {"Name"="FC_2", "Size"=100, "BN"=TRUE, "BN_Params"={"epsilon"=1e-05, "momentum"=0.05}, "Activation"=enum."LReLU", "Has Bias?"=TRUE, "Init_Params"={"Init_Type"=enum."Xavier", "Value"=1.0}, "Custom_Params"=""} ("Layer_Config_Params"), "error in (no error)"=w43, "NN in"=w44) -> ("error out"=w39:errorcluster, "NN out"=w40:T25)  [unwired: 6 in, 1 out]
  n15 = Unbundle By Name(w27) -> ("Dims_Out"=w26:i32)
  n16 = call-poly <vilib>:"NN_Layer_Create.vi"("DropOut_Cfg"=T20 {"Name"="DropOut", "Probability"=0.5}, "error in (no error)"=w39, "NN in"=w40) -> ("error out"=w41:errorcluster, "NN out"=w42:T25)  [unwired: 6 in, 1 out]
  n17 = Bundle By Name(cluster=T13 {"Name"="FC_3", "Size"=10, "BN"=TRUE, "BN_Params"={"epsilon"=1e-05, "momentum"=0.05}, "Activation"=enum."None", "Has Bias?"=TRUE, "Init_Params"={"Init_Type"=enum."Xavier", "Value"=1.0}, "Custom_Params"=""} ("Layer_Config_Params"), "Size"=w26) -> (w52:T13)
  n18 = call-poly <vilib>:"NN_Layer_Create.vi"("FC_Cfg"=w52, "error in (no error)"=w41, "NN in"=w42) -> ("error out"=w54:errorcluster, "NN out"=w55:T25)  [unwired: 6 in, 1 out]
  n19 = call-poly <vilib>:"NN_Layer_Create.vi"("error in (no error)"=w54, "NN in"=w55) -> ("error out"=w34:errorcluster, "NN out"=w66:T25)  [unwired: 7 in, 1 out]
  n20 = call-poly <vilib>:"NN_Set_Loss.vi"("error in (no error)"=w34, "NN in"=w66) -> ("error out"=w33:errorcluster, "NN out"=w35:T25)  [unwired: 8 in]
  n21 = call <vilib>:"NN_Set_Train_Config.vi"("NN_Train_Params"="Train_Params", "error in (no error)"=w33, "NN in"=w35) -> ("error out"=w48:errorcluster, "NN out"=w49:T25)  [unwired: 7 in]
  n22 = Unbundle By Name(w29) -> ("Train"=w30:T23)
  n23 = Unbundle By Name(w29) -> ("Validation"=w59:T23)
  n24 = Unbundle By Name(w29) -> ("Test"=w19:T23)
  n25 = flat-sequence {
    tunnel: [w76] -> w63
    tunnel: w48 -> [_]
    frame #0 {
      n26 = call <vilib>:"High Resolution Relative Seconds.vi"() -> ("relative seconds"=w76:dbl)
    }
  }
  n27 = while {
    shift-right: [w84] -> w60
    shift-left: w48 -> [w77]
    shift-right: [w80] -> w65
    shift-left: w49 -> [w78]
    tunnel: w63 -> [w93]
    tunnel: w30 -> [w83]
    tunnel: w59 -> [w82]
    stop <- w101 stop-if-true
    n28 = Unbundle By Name(w78) -> ("mBatch"=w89:i32)
    n29 = call <vilib>:"NN_Cfg_LR_Decay_Policy.vi"("LR_Decay_Params"="LR Update Policy", "error in (no error)"=w77, "NN in"=w78) -> ("error out"=w96:errorcluster, "NN out"=w102:T25)  [unwired: 7 in]
    n30 = call <vilib>:"High Resolution Relative Seconds.vi"() -> ("relative seconds"=w92:dbl)
    n31 = call <vilib>:"NN_Train.vi"("Train Dataset"=w83, "error in (no error)"=w96, "NN in"=w102) -> ("error out"=w85:errorcluster, "NN out"=w79:T25, "Loss"=w97:sgl)  [unwired: 3 in, 3 out]
    n32 = call <vilib>:"Running_AVG_FIR_Filter.vi"("Numeric"=w97) -> ("Filtered x"=w98:sgl)  [unwired: 10 in]
    n33 = local read "Valid_Error"() -> (w95:sgl)
    n34 = local read "Valid_Loss"() -> (w100:sgl)
    n35 = feedback #1() -> (w103:dbl)  [unwired: 1 in]
    n36 = feedback-in #1(w92) -> ()
    n37 = case shown="True" "Check_Vald" {
      tunnel: w79 -> [w104 w116]
      tunnel: w85 -> [w105 w112]
      tunnel: [w105 w114] -> w84
      tunnel: w82 -> [_ w109]
      tunnel: [w104 w115] -> w80
      frame False {
      }
      frame True {
        n38 = call-poly <vilib>:"NN_Predict.vi"("Dataset"=w109, "error in (no error)"=w112, "NN in"=w116) -> ("error out"=w111:errorcluster, "Predictions"=w110:sgl[][], "NN out"=w113:T25)  [unwired: 6 in]
        n39 = call-poly <vilib>:"NN_Eval.vi"("Dataset"=w109, "error in (no error)"=w111, "Predictions"=w110, "NN in"=w113) -> ("error out"=w114:errorcluster, "NN out"=w115:T25, "NN_Eval_Params"=w108:T35)  [unwired: 4 in, 1 out]
        n40 = Unbundle By Name(w108) -> ("Error"=→"Valid_Error":sgl, "Loss"=→"Valid_Loss":sgl)
      }
    }
    n41 = Subtract(x=w92, y=w93) -> (x-y=→"Time_Elapsed":dbl)
    n42 = Subtract(x=w92, y=w103) -> (x-y=w87:dbl)
    "Train Speed (s/iter)" <- w87
    n43 = Unbundle By Name(w79) -> ("Session Data"=→"Session Data":T4)
    n44 = Divide(x=w89, y=w87) -> (x/y=→"Train Speed (img/s)":dbl)
    n45 = Bundle("Filtered x"=w98, "Valid_Loss"=w100, "Valid_Error"=w95) -> (→"Train Graphs" →"Train/Val_Metrics":T3)  [unwired: 1 in]
    n46 = Compound Arithmetic op=OR(w84, "Stop_Train") -> (w101:bool)
  }
  n47 = call <vilib>:"NN_Destroy_Train.vi"("error in (no error)"=w60, "NN in"=w65) -> ("error out"=w21:errorcluster, "NN out"=w64:T25)  [unwired: 8 in]
  n48 = call-poly <vilib>:"NN_Predict.vi"("Dataset"=w19, "error in (no error)"=w21, "NN in"=w64) -> ("error out"=w20:errorcluster, "Predictions"=w12:sgl[][], "NN out"=w22:T25)  [unwired: 6 in]
  n49 = call-poly <vilib>:"NN_Eval.vi"("Dataset"=w19, "error in (no error)"=w20, "Predictions"=w12, "NN in"=w22) -> ("error out"=w15:errorcluster, "Incrct_Class_idx"=w4:i32[], "NN out"=w17:T25, "NN_Eval_Params"=w1:T35)  [unwired: 4 in]
  n50 = Unbundle By Name(w1) -> ("Error"=→"Test_Error":sgl, "Loss"=→"Test_Loss":sgl)
  n51 = call <vilib>:"NN_to_Categorical.vi"("Prediction"=w12) -> ("Label_Idx"=w18:i32[])  [unwired: 10 in]
  n52 = call "NN_Get_Incorrect_Classified_Imgs(GrayScale)_1D.vi"("Test_Data"=w19, "error in (no error)"=w15, "Predictions"=w12, "MisClassed_idx"=w4) -> ("error out"=w14:errorcluster, "Images(GrayScale)"=→"Incorrectly Classified Imgs":T12[][])  [unwired: 6 in]
  n53 = control-ref of="Confusion Matrix"() -> (w23:refnum<vi>)
  n54 = call-poly <vilib>:"NN_Calc_Confusion_Matrix.vi"("Confusion Matrix (Table) ref."=w23, "error in (no error)"=w14, "Predictions"=w18, "Dataset"=w19) -> ("error out"=w13:errorcluster, "Confusion Matrix (Table)"=→"Confusion Matrix":string[][])  [unwired: 3 in, 3 out]
  n55 = call-poly <vilib>:"NN_Dataset_Destroy.vi"("error in (no error)"=w13, "Datasets_All(In1D_Out1D)"=w29) -> ("error out"=w50:errorcluster)  [unwired: 9 in]
  n56 = Unbundle By Name(w17) -> ("Labels"=→"Labels":string[])
  n57 = while {
    shift-right: [w137] -> w68
    shift-left: w17 -> [w130]
    tunnel: w50 -> [w128]
    tunnel: [w121] -> w67
    stop <- w135 stop-if-true
    n58 = local read "image (28x28px)"() -> (w118:sgl[][])
    n59 = call <vilib>:"High Resolution Relative Seconds.vi"() -> ("relative seconds"=w133:dbl)
    n60 = feedback #2() -> (w134:dbl)  [unwired: 1 in]
    n61 = feedback-in #2(w133) -> ()
    n62 = Subtract(x=w133, y=w134) -> (x-y=w132:dbl)
    "test time(s/img)" <- w132
    n63 = Array Size(array=w118) -> (size(s)=w120:i32[])
    n64 = Reciprocal(x=w132) -> (1/x=→"Test Speed (img/s)":dbl)
    n65 = Multiply Array Elements(1:w120) -> (0:w119:i32)
    n66 = Reshape Array(w118, w119) -> (w117:sgl[])
    n67 = call-poly <vilib>:"NN_Set_Input.vi"("error in (no error)"=w128, "Data_In(1D_SGL)"=w117, "NN In"=w130) -> ("error out"=w127:errorcluster, "NN Out"=w129:T25)  [unwired: 7 in]
    n68 = call <vilib>:"NN_Forward.vi"("error in (no error)"=w127, "NN in"=w129) -> ("error out"=w136:errorcluster, "NN out"=w138:T25)  [unwired: 6 in, 2 out]
    n69 = call <vilib>:"NN_Get_Layer(Last).vi"("error in (no error)"=w136, "NN in"=w138) -> ("error out"=w122:errorcluster, "Last_Layer"=w126:T36, "NN out"=w137:T25)  [unwired: 6 in, 1 out]
    n70 = call <vilib>:"NN_Layer_Get_OutVals_as1D.vi"("error in (no error)"=w122, "Layer"=w126) -> ("error out"=w121:errorcluster, "Out(as1D)"=w125:sgl[][])  [unwired: 8 in]
    n71 = Index Array(array=w125) -> (element=→"Predictions":sgl[])  [unwired: 2 in]
    n72 = Or(x=w121, y="Stop_Test") -> (x .or. y?=w135:bool)
  }
  n73 = case shown="No Error" w50 {
    frame No Error {
      # "Portion of code responsible for drawing interface - Description is not provided as it is out of the scope of the toolkit"
      n74 = call "Empty Picture"() -> ("empty picture"=w141:picture)
      n75 = property on="Draw Digit (280x280 px)" class="Pict"("Value"=w141) -> ()  [unwired: 2 in, 2 out]
      n76 = while {
        shift-right: [w156] -> _
        shift-left: w141 -> [w161]
        shift-right: [w159] -> _
        shift-left: FALSE -> [w160]
        shift-right: [w157] -> _
        shift-left: cluster{"X":i32, "Y":i32} {"X"=0, "Y"=0} ("Mouse Position") -> [w158]
        stop <- w146 stop-if-true
        w143 = sgl 127.0 ("dimension size")
        w147 = 280 ("dimension size")
        w149 = 28
        # "Drawing Interface Loop"
        n77 = event shown="[0] \"Draw Digit (280x280 px)\": Mouse Down" {
          selector: _ -> [_ _ _ _ _ _]
          dyn-events: _ -> [_ _ _ _ _ _]
          timeout: _ -> [_ _ _ _ _ _]
          tunnel: [_ _ _ _ _ "Stop Test"] -> w146
          tunnel: [w186 w193 w204 w207 w210 w213] -> w156
          tunnel: w161 -> [w188 w192 w204 w207 _ w213]
          tunnel: w160 -> [_ w191 _ _ _ _]
          tunnel: [TRUE w191 FALSE FALSE FALSE FALSE] -> w159
          tunnel: w158 -> [_ w190 w202 w206 w209 w212]
          tunnel: [w184 w190 w202 w206 w209 w212] -> w157
          event "Draw Digit (280x280 px)": Mouse Down {
            # "Set the pen position, and draw an initial point or line."
            n78 = event-data() -> ()  [unwired: 1 in, 1 out]
            n79 = property on="Draw Digit (280x280 px)" class="Pict"() -> ("Mouse"=w189:T42)  [unwired: 2 in, 2 out]
            n80 = Unbundle By Name(w189) -> ("Mouse Position"=w184:cluster{"X":i32, "Y":i32})
            n81 = Bundle By Name(cluster=T11 {"Width"=23, "Style"=enum."Solid"} ("Pen Attributes"), "Width"="Pen Width") -> (w180:T11)
            "Pen Attributes" <- w180
            n82 = local read "Pen Color"() -> (w183:u32)
            n83 = call <vilib>:"Move Pen.vi"("new position"=w184, "picture"=w188) -> ("new picture"=w187:picture)  [unwired: 3 in]
            n84 = call <vilib>:"Draw Point.vi"("picture"=w187, "point(x,y)"=w184, "color(black)"=w183, "pen"=w180) -> ("new picture"=w186:picture)  [unwired: 5 in]
          }
          event "Draw Digit (280x280 px)": Mouse Move {
            # "Only draw if a Mouse Down event has occurred, but not a Mouse Up. Then, determine if the user is Drawing a point, a line, or selecting a subset and perform those operations in the case structure."
            n85 = event-data() -> ()  [unwired: 1 in, 1 out]
            n86 = property on="Draw Digit (280x280 px)" class="Pict"() -> ("Mouse"=w194:T42)  [unwired: 2 in, 2 out]
            n87 = case shown="True" w191 {
              tunnel: w192 -> [w195 w201]
              tunnel: w194 -> [_ w200]
              tunnel: [w195 w198] -> w193
              tunnel: w190 -> [_ _]
              frame False {
              }
              frame True {
                n88 = Unbundle By Name(w200) -> ("Mouse Position"=w199:cluster{"X":i32, "Y":i32})
                n89 = local read "Pen Attributes"() -> (w197:T11)
                n90 = call <vilib>:"Draw Line.vi"("picture"=w201, "end point"=w199, "color(black)"="Pen Color", "pen"=w197) -> ("new picture"=w198:picture)  [unwired: 5 in]
              }
            }
          }
          event "Draw Digit (280x280 px)": Mouse Up {
            # "When the user is finished drawing, we complete the operation. The only operation that we need to complete the Select Subset operation."
            n91 = event-data() -> ()  [unwired: 1 in, 1 out]
          }
          event "Draw Digit (280x280 px)": Mouse Leave {
            # "Change to the default cursor when the mouse leaves the picture."
            n92 = event-data() -> ()  [unwired: 1 in, 1 out]
          }
          event "Clear": Value Change {
            # "Erase the picture."
            n93 = event-data() -> ()  [unwired: 1 in, 1 out]
            n94 = call "Empty Picture"() -> ("empty picture"=w210:picture)
          }
          event "Stop Test": Value Change {
            # "Stop the VI."
            n95 = event-data() -> ()  [unwired: 1 in, 1 out]
          }
        }
        "Draw Digit (280x280 px)" <- w156
        n96 = local write "Stop_Test"(w146) -> ()
        n97 = call <vilib>:"Picture to Pixmap.vi"("depth"=8, "rect"=T41 {"left"=0, "top"=0, "right"=280, "bottom"=280}, "picture"=w156) -> ("image data"=w154:T43)  [unwired: 7 in, 1 out]
        n98 = Unbundle By Name(w154) -> ("image"=w152:u8[])
        n99 = Reshape Array(w152, w147, w147) -> (w151:u8[][])
        n100 = Transpose 2D Array(2D array=w151) -> (transposed array=w150:u8[][])
        n101 = for {
          N: w149 -> [_]
          tunnel: w150 -> [w167]
          tunnel: w149 -> [w166]
          tunnel: [w162] -> w148 mode=indexing
          i -> [w165]
          w163 = 10 ("x")
          n102 = Multiply(x=w165, y=w163) -> (x*y=w164:i32)
          n103 = for {
            N: w166 -> [_]
            tunnel: w167 -> [w179]
            tunnel: w164 -> [w178]
            tunnel: w163 -> [w175]
            tunnel: [w168] -> w162 mode=indexing
            i -> [w177]
            w174 = 10 ("length")
            n104 = Multiply(x=w177, y=w175) -> (x*y=w176:i32)
            n105 = Array Subset(array=w179, index (row)=w178, length (row)=w174, index (col)=w176, length (col)=w174) -> (w173:u8[][])
            n106 = To Single Precision Float(number=w173) -> (single precision float=w172:sgl[][])
            n107 = Add Array Elements(numeric array=w172) -> (sum=w171:sgl)
            n108 = Divide(x=w171, y=sgl 100.0 ("x")) -> (x/y=w169:sgl)
            n109 = To Unsigned Byte Integer(number=w169) -> (unsigned 8bit integer=w168:u8)
          }
        }
        n110 = Transpose 2D Array(2D array=w148) -> (transposed array=w144:u8[][])
        n111 = Subtract(x=w144, y=w143) -> (x-y=w145:sgl[][])
        n112 = Divide(x=w145, y=w143) -> (x/y=→"image (28x28px)":sgl[][])
      }
    }
    frame Error {
    }
  }
  n113 = call <vilib>:"NN_Destroy.vi"("Save (T, T, T)"=T21 {"CFG?"=TRUE, "Weights?"=TRUE, "Render?"=TRUE} ("Save_Config"), "error in (no error)"=w67, "NN in"=w68) -> ("error out"=w69:errorcluster)  [unwired: 7 in, 1 out]
  n114 = flat-sequence {
    tunnel: w69 -> [w216]
    frame #0 {
      n115 = call <vilib>:"Simple Error Handler.vi"("error in (no error)"=w216) -> ()  [unwired: 4 in, 5 out]
      n116 = local write "Stop_Test"(FALSE ("Stop_Test")) -> ()
      n117 = Request Deallocation(TRUE ("flag")) -> ()
    }
  }
